vi "全温区自动测试.vi"() -> ()   [LabVIEW 2021]
uses:
  <instrlib>/Keithley DMM6500 DAQ6500 Series/Public/Data/Read (Multiple Points).vi
  <instrlib>/Keithley DMM6500 DAQ6500 Series/Keithley DMM6500 DAQ6500 Series.lvlib
  <instrlib>/TDK-Lambda G Series/TDK-Lambda G Series.lvlib
panel:
  out "数组":T1(array[cluster])
  in  "停止":bool
  out "NTC温度":dbl[](array[numeric])
  out "热电偶温度":dbl[](array[numeric])
  in  "数据储存名":string="分流器测试"
  out "实际电流":dbl
  out "shunt电压":dbl
  in  "shunt电压，实际电流":refnum<visa-resource-name>="USB0::0x05E6::0x6510::04434284::INSTR"
  in  "时间(s)":dbl=1.0 caption="延迟时间(s)"
  in  "设定电流":dbl format="%.1f"
  in  "TDK地址":refnum<visa-resource-name>="TCPIP0::192.168.100.8::inst0::INSTR"
  in  "TC温度读取":refnum<visa-resource-name>="USB0::0x05E6::0x6510::04489851::INSTR"
  in  "数据处理":bool
  in  "停止按钮":bool
  in  "开始测试":bool
  # "嘉晨智能分流器测试"
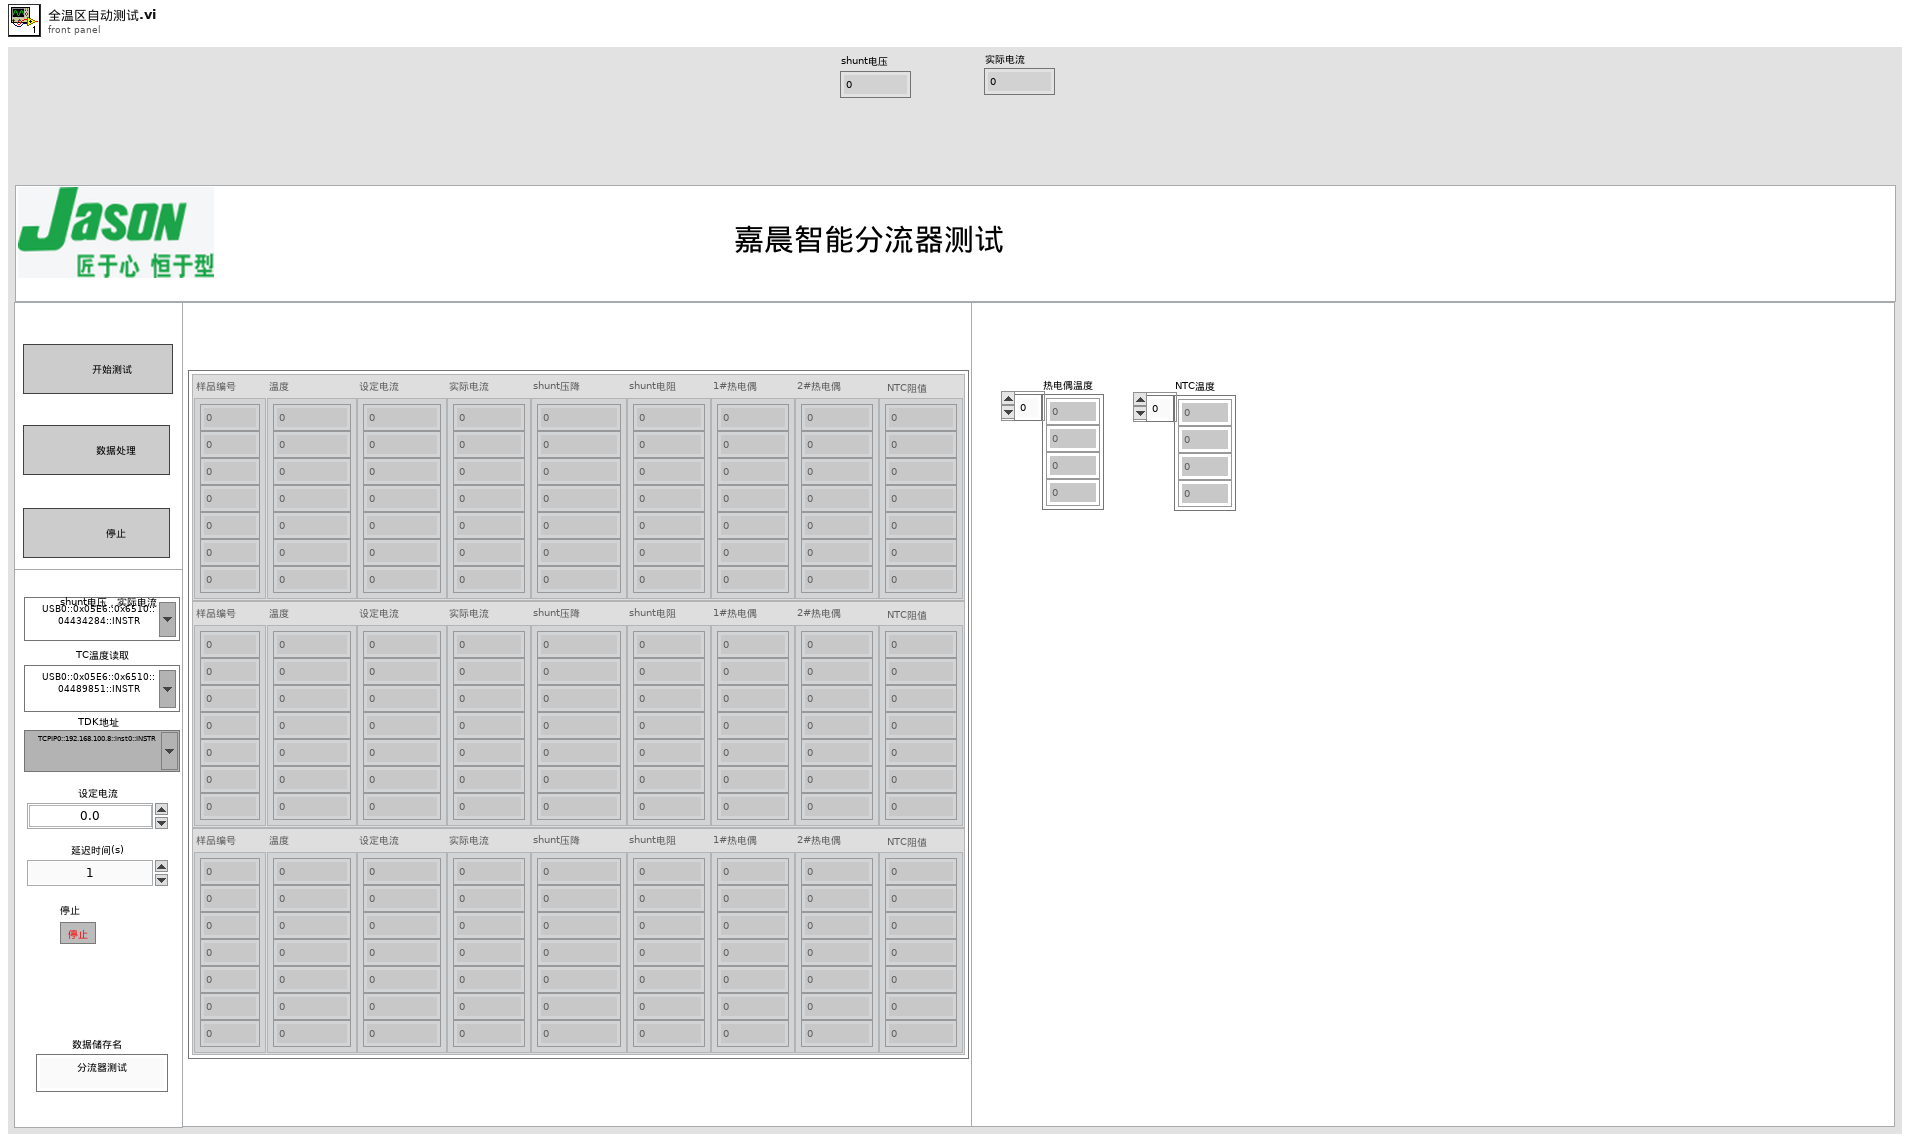
[diagram p1: front panel]
types:
  T1 = cluster{"样品编号":dbl[], "温度":dbl[], "设定电流":dbl[], "实际电流":dbl[], "shunt压降":dbl[], "shunt电阻":dbl[], "1#热电偶":dbl[], "2#热电偶":dbl[], "NTC阻值":dbl[]}[]
  T2 = cluster{dbl[], dbl[], dbl[], dbl[], dbl[], dbl[], dbl[], dbl[], dbl[]}[]
  T3 = typedef "数据显示.ctl" = cluster{"启用":bool, "数据":cluster{"设定电流(A)":dbl, "实际电流(A)":dbl, "电压降(mV)":dbl, "SHUNT电阻(uΩ)":dbl, "1#热电偶温度(℃)":dbl, "2#热电偶温度(℃)":dbl, "NTC温度(℃)":dbl}}
  T4 = cluster{dbl[], dbl[], dbl[], dbl[], dbl[], dbl[], dbl[], dbl[], dbl[]}
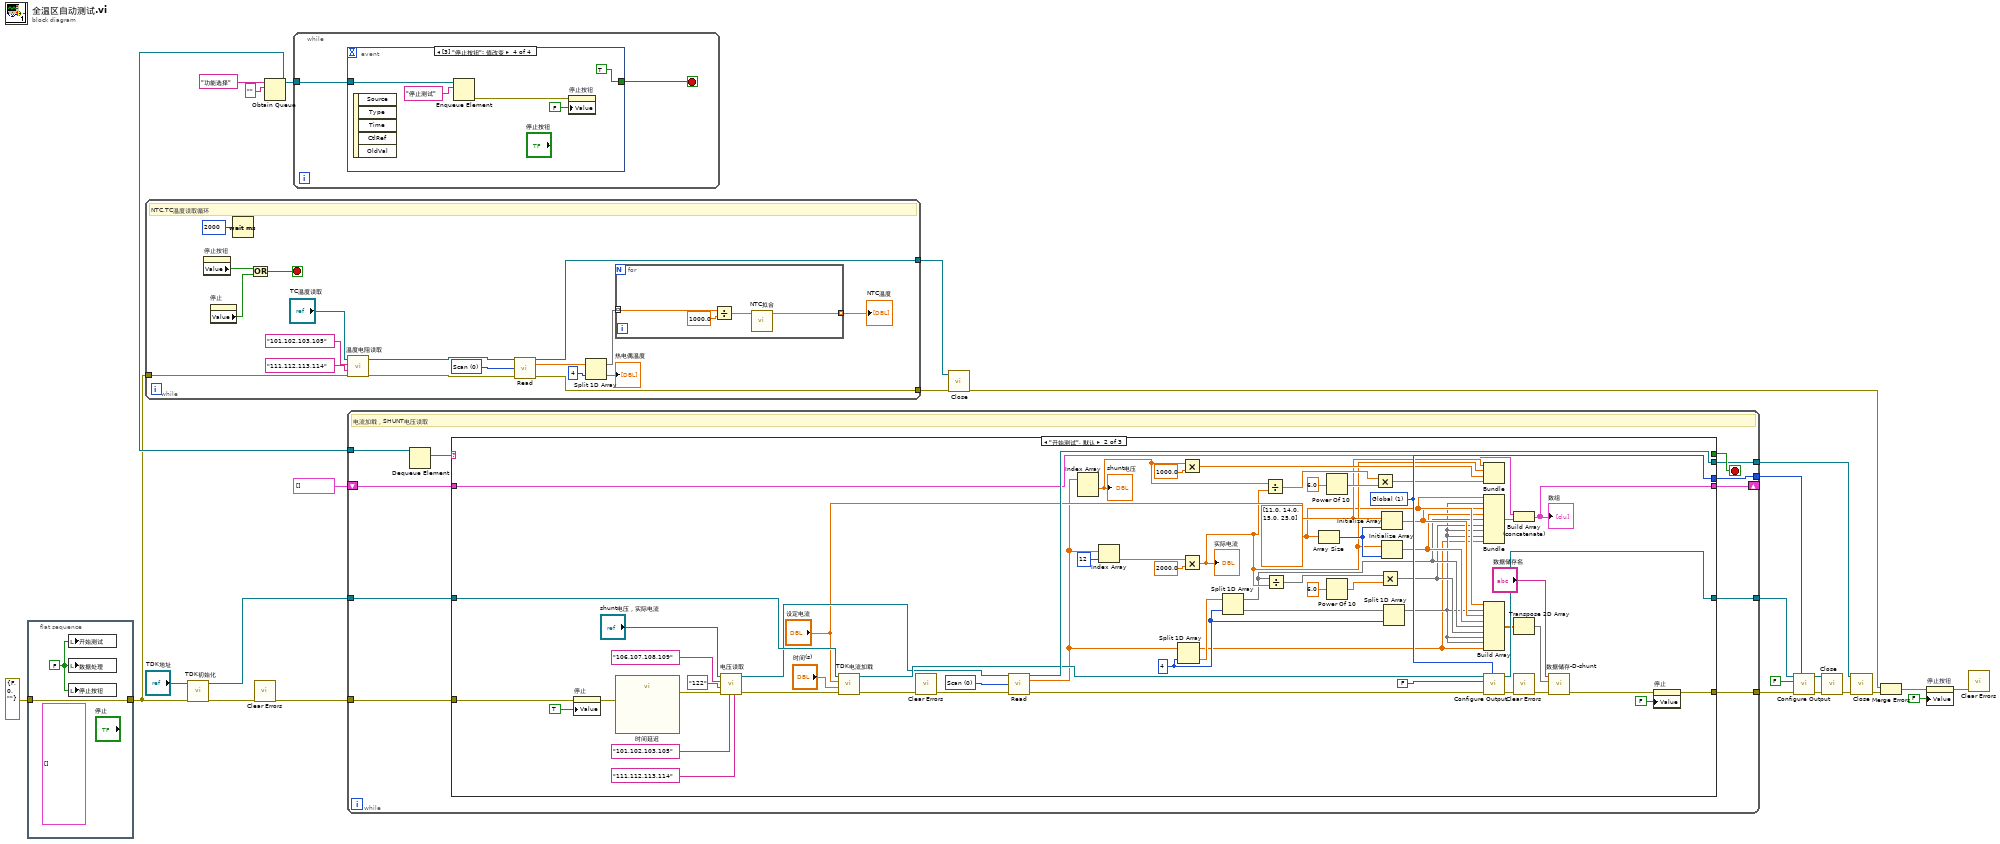
[diagram p0: block diagram]
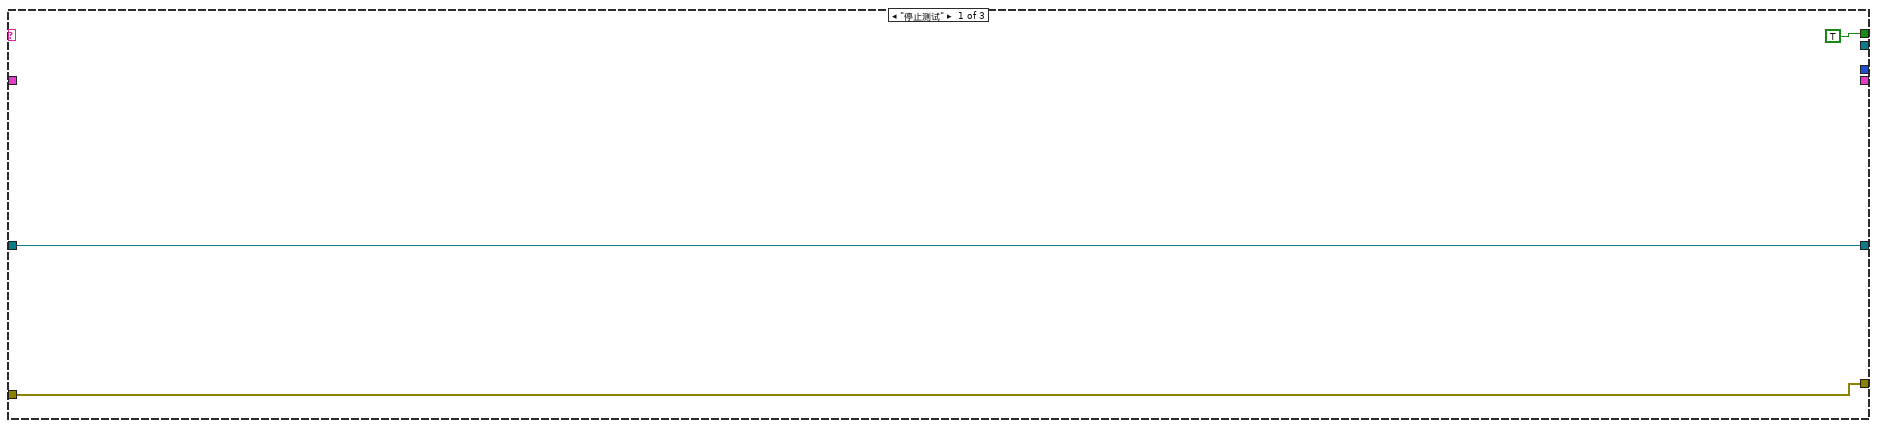
[diagram p2: hidden frame]
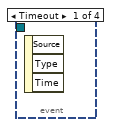
[diagram p4: hidden frame]
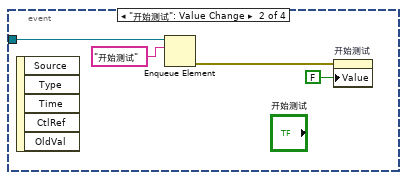
[diagram p5: hidden frame]
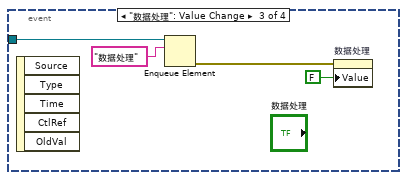
[diagram p6: hidden frame]
diagram:
  n1 = flat-sequence {
    tunnel: errorcluster {"status"=FALSE, "code"=0, "source"=""} ("error in (no error)") -> [w27]
    tunnel: [w27] -> w3
    frame #0 {
      (unwired) T3[] []
      w26 = FALSE ("开始测试")
      n2 = local write "开始测试"(w26) -> ()
      n3 = local write "数据处理"(w26) -> ()
      n4 = local write "停止按钮"(w26) -> ()
    }
  }
  n5 = while {
    tunnel: [w43] -> w22
    tunnel: [w42] -> w21
    tunnel: w3 -> [w35]
    stop <- w28 stop-if-true
    w44 = 0 items=["Scan", "Trigger"] ("Capture Mode(0: Scan)")
    # "NTC,TC温度读取循环"
    n6 = property on="停止按钮" class="Bool (严格)"() -> ("Value"=w30:bool)  [unwired: 2 in, 2 out]
    n7 = property on="停止" class="Bool (严格)"() -> ("Value"=w29:bool)  [unwired: 2 in, 2 out]
    n8 = Wait (ms)(milliseconds to wait=u32 2000 ("等待时间（毫秒）")) -> ()  [unwired: 1 out]
    n9 = Or(x=w30, y=w29) -> (x .or. y?=w28:bool)
    n10 = call "温度电阻读取.vi"("error in (no error)"=w35, "温度通道"="111,112,113,114", "电阻通道"="101,102,103,105", "VISA resource name"="TC温度读取") -> ("error out"=w32:errorcluster, "VISA resource name out"=w31:refnum<visa-resource-name>)  [unwired: 6 in]
    n11 = call-poly <instrlib>:"Read.vi"("VISA resource name"=w31, "Capture Mode(0: Scan)"=w44, "error in (no error)"=w32) -> ("VISA resource name out"=w43:refnum<visa-resource-name>, "Measurements"=w41:dbl[], "error out"=w42:errorcluster)  [unwired: 10 in]
    n12 = Split 1D Array(array=w41, index=4 ("索引")) -> (first subarray=w39:dbl[], second subarray=→"热电偶温度":dbl[])
    n13 = for {
      tunnel: w39 -> [w47] mode=indexing
      tunnel: [w46] -> w37 mode=indexing
      n14 = Divide(x=w47, y=1000.0) -> (x/y=w48:dbl)
      n15 = call "NTC拟合.vi"("NTC电阻"=w48) -> ("NTC温度"=w46:dbl)  [unwired: 10 in]
    }
    "NTC温度" <- w37
  }
  n16 = call "TDK初始化.vi"("error in (no error)"=w3, "TDK地址"="TDK地址") -> ("error out"=w8:errorcluster, "VISA resource name out"=w18:refnum<visa-resource-name>)  [unwired: 8 in]
  n17 = call <vilib>:"Clear Errors.vi"("error in (no error)"=w8) -> ("error out"=w2:errorcluster)  [unwired: 5 in, 1 out]
  n18 = Obtain Queue(name (unnamed)="功能选择" ("名称（未命名）"), element data type="") -> (queue out=w15:refnum<queue>)  [unwired: 3 in, 2 out]
  n19 = while {
    tunnel: w15 -> [w51]
    stop <- w50 stop-if-true
    n20 = event shown="[3] \"停止按钮\": 值改变" {
      selector: _ -> [_ _ _ _]
      dyn-events: _ -> [_ _ _ _]
      timeout: _ -> [_ _ _ _]
      tunnel: w51 -> [_ w55 w58 w64]
      tunnel: [_ _ _ TRUE] -> w50
      event Timeout {
        n21 = event-data() -> ()  [unwired: 1 in, 3 out]
      }
      event "开始测试": Value Change {
        n22 = event-data() -> ()  [unwired: 1 in, 5 out]
        n23 = Enqueue Element(queue=w55, element="开始测试" ("元素")) -> (error out=w52:errorcluster)  [unwired: 2 in, 2 out]
        n24 = property on="开始测试" class="Bool (严格)"(error in=w52, "Value"=FALSE ("开始测试")) -> ()  [unwired: 1 in, 2 out]
      }
      event "数据处理": Value Change {
        n25 = event-data() -> ()  [unwired: 1 in, 5 out]
        n26 = Enqueue Element(queue=w58, element="数据处理" ("元素")) -> (error out=w57:errorcluster)  [unwired: 2 in, 2 out]
        n27 = property on="数据处理" class="Bool (严格)"(error in=w57, "Value"=FALSE ("数据处理")) -> ()  [unwired: 1 in, 2 out]
      }
      event "停止按钮": Value Change {
        n28 = event-data() -> ()  [unwired: 1 in, 5 out]
        n29 = Enqueue Element(queue=w64, element="停止测试" ("元素")) -> (error out=w60:errorcluster)  [unwired: 2 in, 2 out]
        n30 = property on="停止按钮" class="Bool (严格)"(error in=w60, "Value"=FALSE ("停止按钮")) -> ()  [unwired: 1 in, 2 out]
      }
    }
  }
  n31 = while {
    tunnel: w15 -> [w75]
    tunnel: w18 -> [w67]
    tunnel: [w72] -> w12
    tunnel: [w71] -> w17
    tunnel: [w70] -> w14
    tunnel: [w69] -> w7
    tunnel: w2 -> [w68]
    shift-right: [w66] -> _
    shift-left: T2 [] -> [w65]
    stop <- w73 stop-if-true
    # "电流加载，SHUNT电压读取"
    n32 = Dequeue Element(queue=w75) -> (element=w74:string)  [unwired: 2 in, 3 out]
    n33 = case shown="\"开始测试\", 默认" w74 {
      tunnel: [TRUE _ _] -> w73
      tunnel: w67 -> [w77 w138 _]
      tunnel: [w76 w102 _] -> w72
      tunnel: [_ w136 _] -> w71
      tunnel: [w77 w133 _] -> w70
      tunnel: [_ w124 _] -> w69
      tunnel: w68 -> [w76 w109 _]
      tunnel: [_ w88 _] -> w66
      tunnel: w65 -> [_ w89 _]
      frame "停止测试" {
      }
      frame "开始测试", Default {
        w86 = dbl[] [11.0, 14.0, 15.0, 25.0]
        w101 = 4 ("索引")
        w124 = u16 1 items=["Single", "Global"] ("Globalize (0: Single)")
        w131 = 0 items=["Scan", "Trigger"] ("Capture Mode(0: Scan)")
        n34 = property on="停止" class="Bool (严格)"(error in=w109, "Value"=TRUE ("停止")) -> (error out=w106:errorcluster)  [unwired: 1 in, 1 out]
        n35 = call "时间延迟"("error in (no error)"=w106) -> ("error out"=w105:errorcluster)  [unwired: 10 in]
        n36 = call "电压读取.vi"("热电偶通道"="111,112,113,114", "NTC电阻"="101,102,103,105", "error in (no error)"=w105, "实际电流"="122", "电压通道"="106,107,108,109" ("电阻通道"), "VISA resource name"="shunt电压，实际电流") -> ("error out"=w112:errorcluster, "VISA resource name out"=w111:refnum<visa-resource-name>)  [unwired: 4 in]
        n37 = call "TDK电流加载.vi"("error in (no error)"=w112, "时间(s)"="时间(s)", "电流"="设定电流", "VISA resource name"=w138) -> ("error out"=w129:errorcluster, "VISA resource name out"=w134:refnum<visa-resource-name>)  [unwired: 6 in]
        n38 = call <vilib>:"Clear Errors.vi"("error in (no error)"=w129) -> ("error out"=w128:errorcluster)  [unwired: 5 in, 1 out]
        n39 = call-poly <instrlib>:"Read.vi"("VISA resource name"=w111, "Capture Mode(0: Scan)"=w131, "error in (no error)"=w128) -> ("VISA resource name out"=w136:refnum<visa-resource-name>, "Measurements"=w97:dbl[], "error out"=w135:errorcluster)  [unwired: 10 in]
        n40 = Index Array(array=w97) -> (element #1=w121:dbl)  [unwired: 2 in, 1 out]
        "shunt电压" <- w121
        n41 = Index Array(array=w97, index=12 ("索引")) -> (element=w94:dbl)
        n42 = Split 1D Array(array=w97, index=w101) -> (first subarray=w80:dbl[], second subarray=w100:dbl[])
        n43 = Multiply(x=w121, y=1000.0) -> (x*y=w120:dbl)
        n44 = Multiply(x=w94, y=2000.0) -> (x*y=w93:dbl)
        "实际电流" <- w93
        n45 = Split 1D Array(array=w100, index=w101) -> (first subarray=w83:dbl[], second subarray=w99:dbl[])
        n46 = Divide(x=w121, y=w93) -> (x/y=w117:dbl)
        n47 = Divide(x=w83, y=w93) -> (x/y=w90:dbl[])
        n48 = Array Size(array=w86) -> (size(s)=w95:i32)
        n49 = Power Of 10(x=6.0) -> (10^x=w118:dbl)
        n50 = Power Of 10(x=6.0) -> (10^x=w91:dbl)
        n51 = Multiply(x=w117, y=w118) -> (x*y=w116:dbl)
        n52 = Multiply(x=w90, y=w91) -> (x*y=w82:dbl[])
        n53 = Initialize Array("设定电流", w95) -> (w85:dbl[])
        n54 = Initialize Array(w93, w95) -> (w84:dbl[])
        n55 = Split 1D Array(array=w99, index=w101) -> (first subarray=w81:dbl[])  [unwired: 1 out]
        n56 = Bundle("设定电流"="设定电流", w93, w120, w116) -> ()  [unwired: 1 in, 1 out]
        n57 = Bundle(w86, w81, w85, w84, w83, w82, w81, w81, w80) -> (w87:T4)  [unwired: 1 in]
        n58 = Build Array(w86, w81, w85, w84, w83, w82, w81, w81, w80) -> (w79:dbl[][])
        n59 = call <instrlib>:"Configure Output.vi"("Globalize (0: Single)"=w124, "error in (no error)"=w135, "Enable Output (False)"=FALSE, "VISA resource name"=w134) -> ("error out"=w127:errorcluster, "VISA resource name out"=w133:refnum<visa-resource-name>)  [unwired: 6 in]
        n60 = Build Array (concatenate)(w89, w87) -> (w88:T2)
        "数组" <- w88
        n61 = Transpose 2D Array(2D array=w79) -> (transposed array=w123:dbl[][])
        n62 = call <vilib>:"Clear Errors.vi"("error in (no error)"=w127) -> ("error out"=w126:errorcluster)  [unwired: 5 in, 1 out]
        n63 = call "数据储存-D-shunt.vi"("错误输入"=w126, "2D data"=w123, "数据储存"="数据储存名") -> ("error out"=w103:errorcluster)  [unwired: 8 in]
        n64 = property on="停止" class="Bool (严格)"(error in=w103, "Value"=FALSE ("停止")) -> (error out=w102:errorcluster)  [unwired: 1 in, 1 out]
      }
      frame "数据处理" {
      }
    }
  }
  n65 = call <instrlib>:"Close.vi"("error in (no error)"=w21, "VISA resource name"=w22) -> ("error out"=w23:errorcluster)  [unwired: 9 in]
  n66 = call <instrlib>:"Configure Output.vi"("Globalize (0: Single)"=w7, "error in (no error)"=w12, "Enable Output (False)"=FALSE, "VISA resource name"=w14) -> ("error out"=w11:errorcluster, "VISA resource name out"=w13:refnum<visa-resource-name>)  [unwired: 6 in]
  n67 = call <instrlib>:"Close.vi"("error in (no error)"=w11, "VISA resource name"=w13) -> ("error out"=w16:errorcluster)  [unwired: 9 in]
  n68 = call <instrlib>:"Close.vi"("error in (no error)"=w16, "VISA resource name"=w17) -> ("error out"=w9:errorcluster)  [unwired: 9 in]
  n69 = Merge Errors(w23, w9) -> (w6:errorcluster)
  n70 = property on="停止按钮" class="Bool (严格)"(error in=w6, "Value"=FALSE ("停止按钮")) -> (error out=w5:errorcluster)  [unwired: 1 in, 1 out]
  n71 = call <vilib>:"Clear Errors.vi"("error in (no error)"=w5) -> ()  [unwired: 5 in, 2 out]
